vi "IsZOffsetValid.vi"(7 "Joystick Offset In":T1) -> (1 "IsZOffsetValid?":bool, 3 "Joystick Offset":T1)   [LabVIEW 2014]
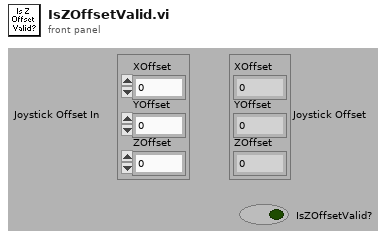
[diagram p1: front panel]
types:
  T1 = cluster{"XOffset":i32, "YOffset":i32, "ZOffset":i32}
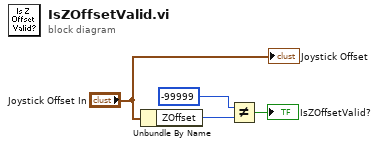
[diagram p0: block diagram]
diagram:
  n1 = Unbundle By Name("Joystick Offset In") -> ("ZOffset"=w3:i32)
  n2 = Not Equal?(x=-99999 ("XRelPos"), y=w3) -> (x != y?=→"IsZOffsetValid?":bool)
  "Joystick Offset" <- "Joystick Offset In"
